vi "Create Oneof Protobuf To Field Name.vi"(8 "error in (no error)":errorcluster, 10 "message element metadata":T1={"Field Name"="nested_message_2", "Embedded Message Name"="echo_array_NestedMessage2", "Protobuf Index"=3, "MessageElementType"=enum."MessageValue", "Repeated"=FALSE, "Is in Oneof"=TRUE, "Oneof Container Name"="echo_array_NestedMessage_union"}, 11 "class in":refnum<vi>) -> (0 "error out":errorcluster, 3 "class out":refnum<vi>)   [LabVIEW 2019, in "gRPC Template Creation Utility.lvlib"]
uses:
  gRPC Template Creation Utility.lvlib
  <vilib>/Utility/traverseref.llb/VI Scripting - Traverse.lvlib
  <vilib>/Utility/traverseref.llb/TRef TravTarget.ctl
  TypeDefs/Message Element Type.ctl
  TypeDefs/Message Element Metadata (Scripting).ctl
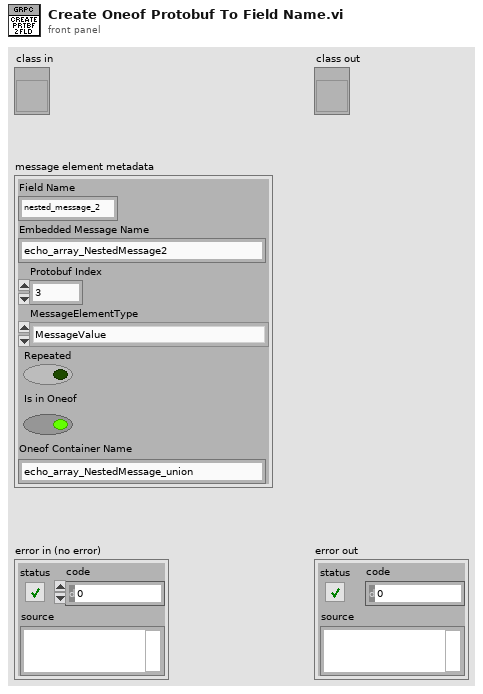
[diagram p1: front panel]
types:
  T1 = typedef "gRPC Template Creation Utility.lvlib/Message Element Metadata (Scripting).ctl" = cluster{"Field Name":string, "Embedded Message Name":string, "Protobuf Index":i32, "MessageElementType":T2, "Repeated":bool, "Is in Oneof":bool, "Oneof Container Name":string}
  T2 = typedef "gRPC Template Creation Utility.lvlib/Message Element Type.ctl" = enum32{"Int32Value", "FloatValue", "DoubleValue", "BoolValue", "StringValue", "MessageValue", "Int64Value", "UInt32Value", "UInt64Value", "EnumValue", "Bytes", "Fixed64", "Fixed32", "SFixed64", "SFixed32", "SInt64", "SInt32"}
  T3 = typedef "TRef TravTarget.ctl" = enum16{"FP", "BD", "Other"}
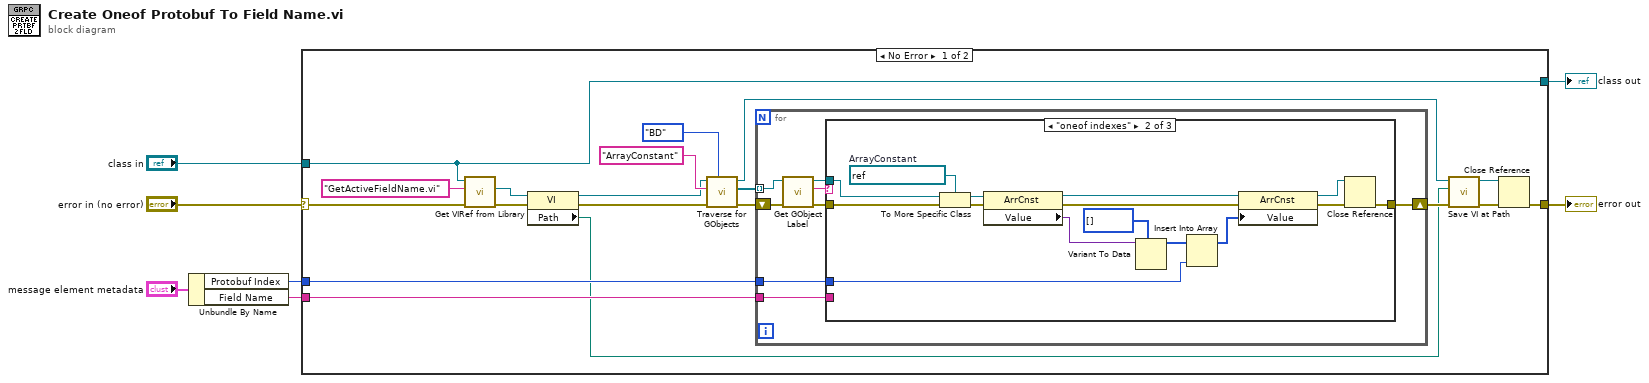
[diagram p0: block diagram]
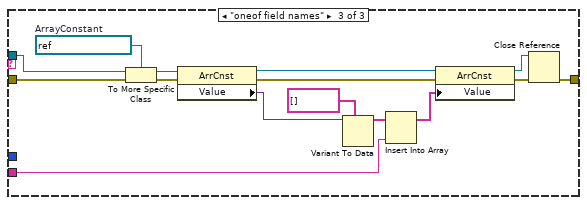
[diagram p3: hidden frame]
diagram:
  n1 = Unbundle By Name("message element metadata") -> ("Protobuf Index"=w1:i32, "Field Name"=w2:string)
  n2 = case shown="No Error" "error in (no error)" {
    selector: "error in (no error)" -> [w14 w66]
    tunnel: "class in" -> [w15 w67]
    tunnel: w1 -> [w24 _]
    tunnel: w2 -> [w23 _]
    tunnel: [w8 w66] -> w6
    tunnel: [w15 w67] -> w5
    frame No Error {
      n3 = call "Get VIRef from Library.vi"("error in (no error)"=w14, "item name"="GetActiveFieldName.vi", "library in"=w15) -> ("error out"=w17:errorcluster, "vi"=w16:refnum<vi>)  [unwired: 5 in, 2 out]
      n4 = property class="VI"(reference=w16, error in=w17) -> (reference out=w11:refnum<vi>, error out=w12:errorcluster, "Path"=w18:path)
      n5 = call <vilib>:"Traverse for GObjects.vi"("Traverse Target"=TRef_TravTarget."BD", "error in (no error)"=w12, "Class Name"="ArrayConstant", "VI Refnum"=w11) -> ("error out"=w22:errorcluster, "References"=w26:refnum<vi>[], "dup VI Refnum"=w20:refnum<vi>)  [unwired: 4 in, 1 out]
      n6 = for {
        tunnel: w26 -> [w34] mode=indexing
        tunnel: w24 -> [w31]
        tunnel: w23 -> [w30]
        shift-right: [w29] -> w19
        shift-left: w22 -> [w27]
        n7 = call <vilib>:"Get GObject Label.vi"("error in (no error)"=w27, "GObject"=w34) -> ("error out"=w28:errorcluster, "Object Label"=w33:string, "dup GObject"=w32:refnum<vi>)  [unwired: 5 in, 2 out]
        n8 = case shown="\"oneof indexes\"" w33 {
          tunnel: w32 -> [_ w50 w57]
          tunnel: w31 -> [_ w44 _]
          tunnel: w30 -> [_ _ w56]
          tunnel: [w35 w38 w53] -> w29
          tunnel: w28 -> [w35 w36 w52]
          frame Default {
          }
          frame "oneof indexes" {
            w49 = refnum<vi> refnum  # ArrayConstant
            n9 = To More Specific Class(target class=w49, reference=w50, error in=w36) -> (specific class reference=w48:refnum<vi>, error out=w42:errorcluster)
            n10 = property class="ArrCnst"(reference=w48, error in=w42) -> (reference out=w47:refnum<vi>, error out=w41:errorcluster, "Value"=w46:variant)
            n11 = Variant To Data(type=i32[] [], Variant=w46) -> (data=w37:i32[])  [unwired: 1 in, 1 out]
            n12 = Insert Into Array(array=w37, new element=w44) -> (w43:i32[])  [unwired: 1 in]
            n13 = property class="ArrCnst"(reference=w47, error in=w41, "Value"=w43) -> (reference out=w39:refnum<vi>, error out=w40:errorcluster)
            n14 = Close Reference(reference=w39, error in (no error)=w40) -> (error out=w38:errorcluster)
          }
          frame "oneof field names" {
            w65 = refnum<vi> refnum  # ArrayConstant
            n15 = To More Specific Class(target class=w65, reference=w57, error in=w52) -> (specific class reference=w64:refnum<vi>, error out=w59:errorcluster)
            n16 = property class="ArrCnst"(reference=w64, error in=w59) -> (reference out=w63:refnum<vi>, error out=w58:errorcluster, "Value"=w62:variant)
            n17 = Variant To Data(type=string[] [], Variant=w62) -> (data=w51:string[])  [unwired: 1 in, 1 out]
            n18 = Insert Into Array(array=w51, new element=w56) -> (w60:string[])  [unwired: 1 in]
            n19 = property class="ArrCnst"(reference=w63, error in=w58, "Value"=w60) -> (reference out=w55:refnum<vi>, error out=w54:errorcluster)
            n20 = Close Reference(reference=w55, error in (no error)=w54) -> (error out=w53:errorcluster)
          }
        }
      }
      n21 = call "Save VI at Path.vi"("error in (no error)"=w19, "Path"=w18, "VI in"=w20) -> ("error out"=w10:errorcluster, "VI out"=w9:refnum<vi>)  [unwired: 6 in, 1 out]
      n22 = Close Reference(reference=w9, error in (no error)=w10) -> (error out=w8:errorcluster)
    }
    frame Error {
    }
  }
  "error out" <- w6
  "class out" <- w5
